vi "teste.vi"(9 "Numeric":dbl) -> (1 "Boolean":bool)   [LabVIEW 2023]
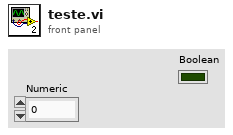
[diagram p1: front panel]
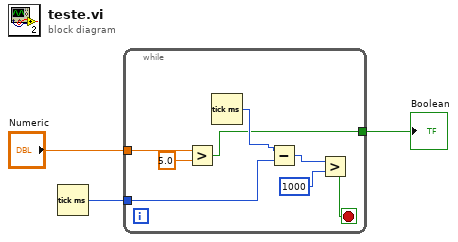
[diagram p0: block diagram]
diagram:
  n1 = Tick Count (ms)() -> (millisecond timer value=w3:u32)
  n2 = while {
    tunnel: w3 -> [w9]
    tunnel: "Numeric" -> [w6]
    tunnel: [w4] -> w1
    stop <- w11 stop-if-true
    n3 = Greater?(x=w6, y=5.0) -> (0:w4:bool)
    n4 = Tick Count (ms)() -> (millisecond timer value=w10:u32)
    n5 = Subtract(x=w10, y=w9) -> (x-y=w8:u32)
    n6 = Greater?(x=w8, y=u32 1000) -> (0:w11:bool)
  }
  "Boolean" <- w1
